vi "changeMode.vi"(8 "error in (no error)":errorcluster, 10 "Measurement":T1 caption="Measurement Function (0: Current)" items=["Current", "Charge", "Voltage", "Resistance"], 11 "Electrometer in":refnum<class "Electrometer.lvclass">) -> (0 "error out":errorcluster, 3 "Electrometer out":refnum<class "Electrometer.lvclass">)   [LabVIEW 2016, in "Electrometer.lvclass"]
uses:
  Electrometer.lvclass
  Modes.ctl
  State/State.lvclass
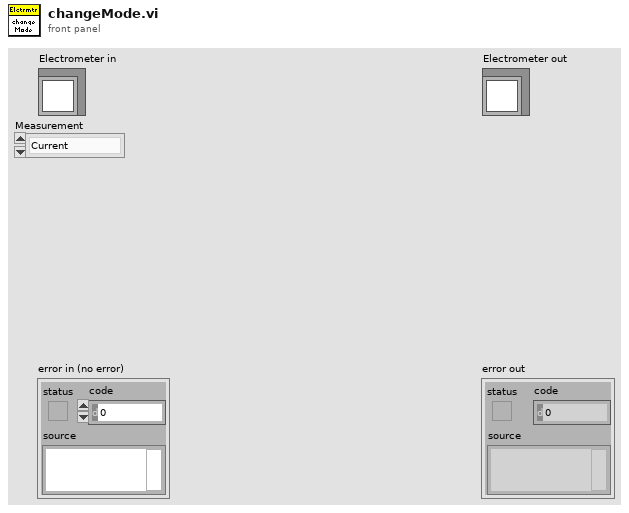
[diagram p1: front panel]
types:
  T1 = typedef "Electrometer.lvclass/Modes.ctl" = i32
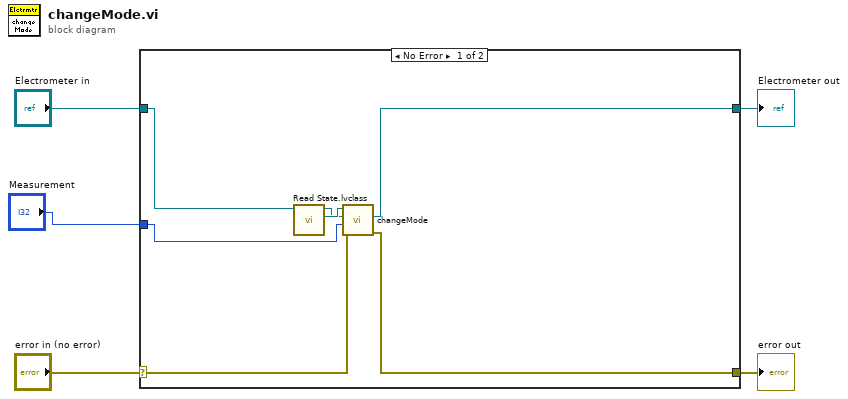
[diagram p0: block diagram]
diagram:
  n1 = case shown="No Error" "error in (no error)" {
    selector: "error in (no error)" -> [w11 w14]
    tunnel: [w10 w14] -> w4
    tunnel: [w6 w13] -> w2
    tunnel: "Electrometer in" -> [w8 w13]
    tunnel: "Measurement" -> [w9 _]
    frame No Error {
      n2 = call-dynamic "Read State.lvclass.vi"("Electrometer in"=w8) -> ("State.lvclass"=w12:refnum<class "State.lvclass">, "Electrometer out"=w7:refnum<class "Electrometer.lvclass">)  [unwired: 8 in, 1 out]
      n3 = call-dynamic "changeMode.vi"("error in (no error)"=w11, "Mode"=w9, "Electrometer in"=w7, "State in"=w12) -> ("error out"=w10:errorcluster, "Electrometer out"=w6:refnum<class "Electrometer.lvclass">)  [unwired: 5 in, 1 out]
    }
    frame Error {
    }
  }
  "error out" <- w4
  "Electrometer out" <- w2
